vi "Bi-mode_VI_modified.vi"() -> ()   [LabVIEW 2014]
doc: "This VI demonstrates the individual configuration of settings in I/W, W/I, and continuous operation modes.\n\nThis VI is not meant to be used with infusion-only models. \n\nNotes:\n(1) If continuous mode is selected, infuse volumes/rates will be used."
uses:
  <instrlib>/KD Scientific 2XX Series/KD Scientific 2XX Series.lvlib
panel:
  out "Units":string
  out "Delivered Volume":dbl
  in  "stop":bool
  out "Status":T1
  in  "Baud Rate (9600)":u32(ring)=9600 items=["300"=300, "1200"=1200, "2400"=2400, "4800"=4800, "9600"=9600]
  in  "Withdrawal Settings":T2={"Flow Rate (5)"=5.0, "Volume (10)"=10.0, "Volume Units (ml)"=enum."milliliters (ml)", "Rate Units (ml/min.)"=enum."milliliters per minute (ml/min.)"} {"Volume (10)" format="%#.3g"}
  in  "Diameter (8.75 mm)":dbl=8.75
  in  "Infusion Settings":T2={"Flow Rate (5)"=5.0, "Volume (10)"=10.0, "Volume Units (ml)"=enum."milliliters (ml)", "Rate Units (ml/min.)"=enum."milliliters per minute (ml/min.)"}
  in  "Operation Mode (Infuse)":u16(ring) items=["Infuse", "Withdraw", "Infuse-Withdraw", "Withdraw-Infuse", "Continuous"]
  in  "Address (0)":i32 format="%0.0f"
  in  "error in (no error)":errorcluster
  in  "VISA resource name":refnum<visa-resource-name>="COM1"
  # "© 2005 National Instruments Corporation.  ALL RIGHTS RESERVED."
  # "RS-232 Settings"
  # "General Settings"
  # "Pump Status"
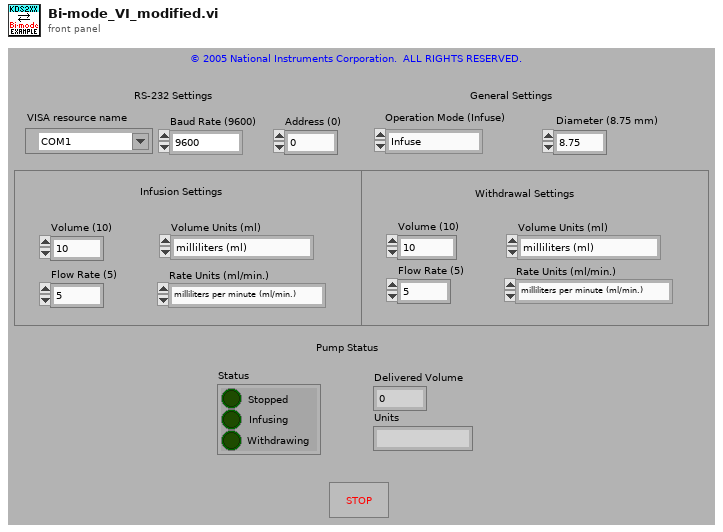
[diagram p1: front panel]
types:
  T1 = cluster{"Stopped":bool, "Infusing":bool, "Withdrawing":bool}
  T2 = cluster{"Flow Rate (5)":dbl, "Volume (10)":dbl, "Volume Units (ml)":enum16{"milliliters (ml)", "microliters (ul)"}, "Rate Units (ml/min.)":enum16{"milliliters per minute (ml/min.)", "milliliters per hour (ml/hr.)", "microliters per minute (ul/min.)", "microliters per hour (ul/hr.)"}}
  T3 = enum16{"milliliters per minute (ml/min.)", "milliliters per hour (ml/hr.)", "microliters per minute (ul/min.)", "microliters per hour (ul/hr.)"}
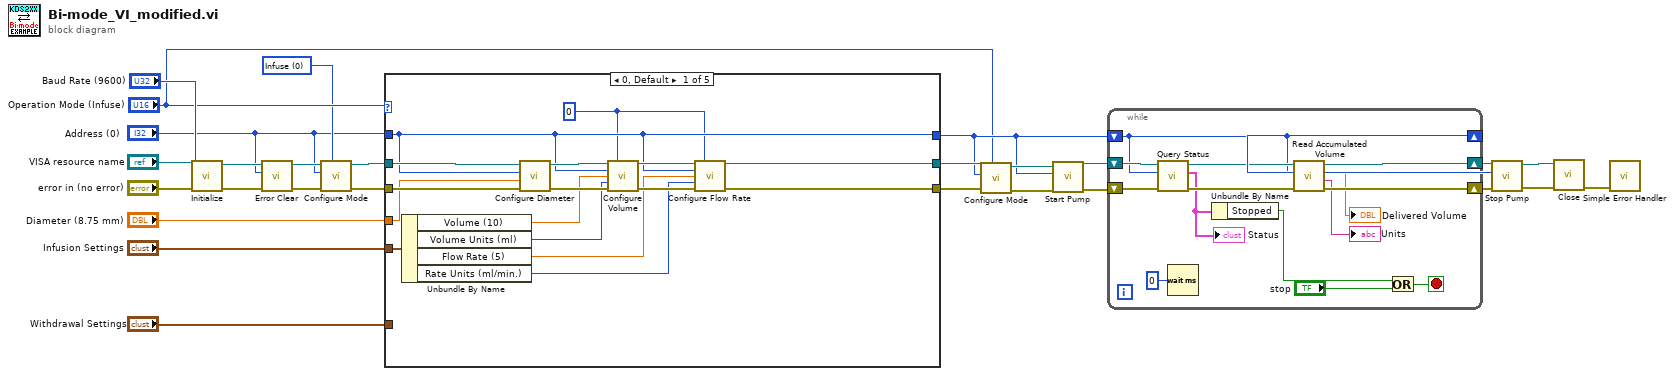
[diagram p0: block diagram]
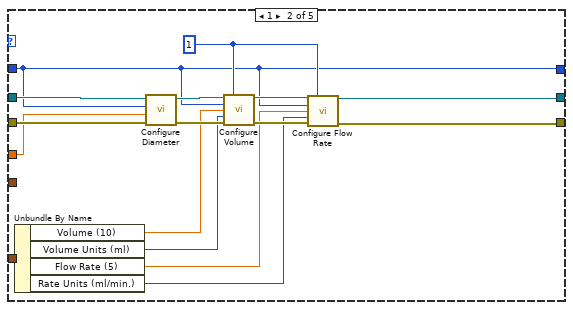
[diagram p2: hidden frame]
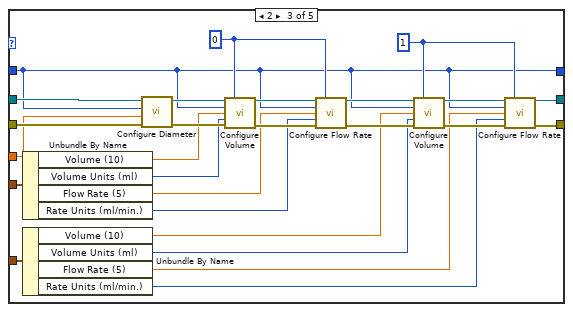
[diagram p3: hidden frame]
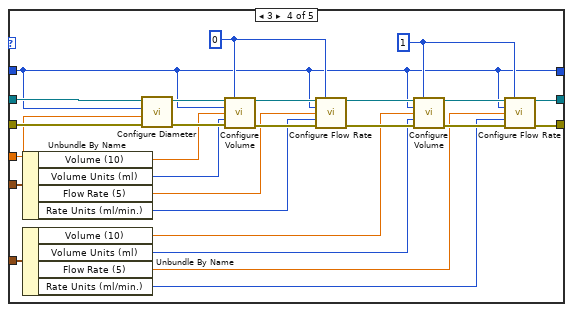
[diagram p4: hidden frame]
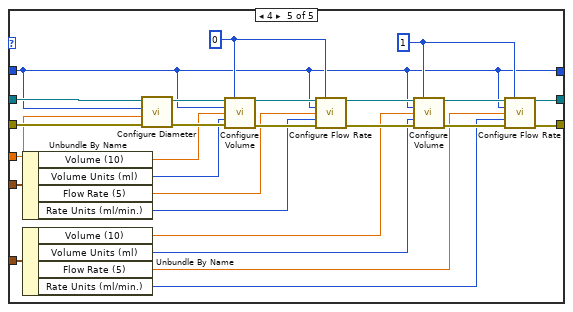
[diagram p5: hidden frame]
diagram:
  w6 = u16 0 items=["Infuse", "Withdraw", "Infuse-Withdraw", "Withdraw-Infuse", "Continuous"] ("Mode (infuse)")
  n1 = call <instrlib>:"Initialize.vi"("error in (no error)"="error in (no error)", "Baud Rate (9600)"="Baud Rate (9600)", "VISA resource name"="VISA resource name") -> ("error out"=w3:errorcluster, "VISA resource name out"=w2:refnum<visa-resource-name>)  [unwired: 7 in]
  n2 = call <instrlib>:"Error Clear.vi"("error in (no error)"=w3, "Address (0)"="Address (0)", "VISA resource name"=w2) -> ("error out"=w4:errorcluster, "VISA resource name out"=w5:refnum<visa-resource-name>)  [unwired: 6 in, 1 out]
  n3 = call <instrlib>:"Configure Mode.vi"("Mode (infuse)"=w6, "error in (no error)"=w4, "Address (0)"="Address (0)", "VISA resource name"=w5) -> ("error out"=w8:errorcluster, "VISA resource name out"=w7:refnum<visa-resource-name>)  [unwired: 6 in]
  n4 = case shown="0, Default" "Operation Mode (Infuse)" {
    tunnel: "Infusion Settings" -> [w38 _ w86 w112 w138]
    tunnel: "Withdrawal Settings" -> [_ w60 w85 w111 w137]
    tunnel: w7 -> [w44 w59 w84 w110 w136]
    tunnel: w8 -> [w43 w55 w83 w109 w135]
    tunnel: "Diameter (8.75 mm)" -> [w37 w51 w66 w92 w118]
    tunnel: [w36 w45 w61 w87 w113] -> w10
    tunnel: "Address (0)" -> [w36 w45 w61 w87 w113]
    tunnel: [w31 w56 w63 w89 w115] -> w14
    tunnel: [w30 w52 w62 w88 w114] -> w13
    frame 0, Default {
      w29 = 0
      n5 = Unbundle By Name(w38) -> ("Volume (10)"=w35:dbl, "Volume Units (ml)"=w34:enum16{"milliliters (ml)", "microliters (ul)"}, "Flow Rate (5)"=w33:dbl, "Rate Units (ml/min.)"=w32:T3)
      n6 = call <instrlib>:"Configure Diameter.vi"("error in (no error)"=w43, "Diameter (8.75 mm)"=w37, "Address (0)"=w36, "VISA resource name"=w44) -> ("error out"=w41:errorcluster, "VISA resource name out"=w42:refnum<visa-resource-name>)  [unwired: 6 in]
      n7 = call <instrlib>:"Configure Volume.vi"("VISA resource name"=w42, "Mode (infuse)"=w29, "Address (0)"=w36, "Volume (100)"=w35, "Units (0: milliliters)"=w34, "error in (no error)"=w41) -> ("VISA resource name out"=w40:refnum<visa-resource-name>, "error out"=w39:errorcluster)  [unwired: 8 in]
      n8 = call <instrlib>:"Configure Flow Rate.vi"("VISA resource name"=w40, "Mode (infuse)"=w29, "Address (0)"=w36, "Flow Rate (5)"=w33, "Units (0: milliliters per minute)"=w32, "error in (no error)"=w39) -> ("VISA resource name out"=w31:refnum<visa-resource-name>, "error out"=w30:errorcluster)  [unwired: 8 in]
    }
    frame 1 {
      w46 = 1
      n9 = Unbundle By Name(w60) -> ("Volume (10)"=w50:dbl, "Volume Units (ml)"=w49:enum16{"milliliters (ml)", "microliters (ul)"}, "Flow Rate (5)"=w48:dbl, "Rate Units (ml/min.)"=w47:T3)
      n10 = call <instrlib>:"Configure Diameter.vi"("error in (no error)"=w55, "Diameter (8.75 mm)"=w51, "Address (0)"=w45, "VISA resource name"=w59) -> ("error out"=w54:errorcluster, "VISA resource name out"=w58:refnum<visa-resource-name>)  [unwired: 6 in]
      n11 = call <instrlib>:"Configure Volume.vi"("VISA resource name"=w58, "Mode (infuse)"=w46, "Address (0)"=w45, "Volume (100)"=w50, "Units (0: milliliters)"=w49, "error in (no error)"=w54) -> ("VISA resource name out"=w57:refnum<visa-resource-name>, "error out"=w53:errorcluster)  [unwired: 8 in]
      n12 = call <instrlib>:"Configure Flow Rate.vi"("VISA resource name"=w57, "Mode (infuse)"=w46, "Address (0)"=w45, "Flow Rate (5)"=w48, "Units (0: milliliters per minute)"=w47, "error in (no error)"=w53) -> ("VISA resource name out"=w56:refnum<visa-resource-name>, "error out"=w52:errorcluster)  [unwired: 8 in]
    }
    frame 2 {
      w64 = 1
      w65 = 0
      n13 = Unbundle By Name(w86) -> ("Volume (10)"=w74:dbl, "Volume Units (ml)"=w73:enum16{"milliliters (ml)", "microliters (ul)"}, "Flow Rate (5)"=w72:dbl, "Rate Units (ml/min.)"=w71:T3)
      n14 = Unbundle By Name(w85) -> ("Volume (10)"=w70:dbl, "Volume Units (ml)"=w69:enum16{"milliliters (ml)", "microliters (ul)"}, "Flow Rate (5)"=w68:dbl, "Rate Units (ml/min.)"=w67:T3)
      n15 = call <instrlib>:"Configure Diameter.vi"("error in (no error)"=w83, "Diameter (8.75 mm)"=w66, "Address (0)"=w61, "VISA resource name"=w84) -> ("error out"=w78:errorcluster, "VISA resource name out"=w82:refnum<visa-resource-name>)  [unwired: 6 in]
      n16 = call <instrlib>:"Configure Volume.vi"("VISA resource name"=w82, "Mode (infuse)"=w65, "Address (0)"=w61, "Volume (100)"=w74, "Units (0: milliliters)"=w73, "error in (no error)"=w78) -> ("VISA resource name out"=w81:refnum<visa-resource-name>, "error out"=w77:errorcluster)  [unwired: 8 in]
      n17 = call <instrlib>:"Configure Flow Rate.vi"("VISA resource name"=w81, "Mode (infuse)"=w65, "Address (0)"=w61, "Flow Rate (5)"=w72, "Units (0: milliliters per minute)"=w71, "error in (no error)"=w77) -> ("VISA resource name out"=w80:refnum<visa-resource-name>, "error out"=w76:errorcluster)  [unwired: 8 in]
      n18 = call <instrlib>:"Configure Volume.vi"("VISA resource name"=w80, "Mode (infuse)"=w64, "Address (0)"=w61, "Volume (100)"=w70, "Units (0: milliliters)"=w69, "error in (no error)"=w76) -> ("VISA resource name out"=w79:refnum<visa-resource-name>, "error out"=w75:errorcluster)  [unwired: 8 in]
      n19 = call <instrlib>:"Configure Flow Rate.vi"("VISA resource name"=w79, "Mode (infuse)"=w64, "Address (0)"=w61, "Flow Rate (5)"=w68, "Units (0: milliliters per minute)"=w67, "error in (no error)"=w75) -> ("VISA resource name out"=w63:refnum<visa-resource-name>, "error out"=w62:errorcluster)  [unwired: 8 in]
    }
    frame 3 {
      w90 = 1
      w91 = 0
      n20 = Unbundle By Name(w112) -> ("Volume (10)"=w100:dbl, "Volume Units (ml)"=w99:enum16{"milliliters (ml)", "microliters (ul)"}, "Flow Rate (5)"=w98:dbl, "Rate Units (ml/min.)"=w97:T3)
      n21 = Unbundle By Name(w111) -> ("Volume (10)"=w96:dbl, "Volume Units (ml)"=w95:enum16{"milliliters (ml)", "microliters (ul)"}, "Flow Rate (5)"=w94:dbl, "Rate Units (ml/min.)"=w93:T3)
      n22 = call <instrlib>:"Configure Diameter.vi"("error in (no error)"=w109, "Diameter (8.75 mm)"=w92, "Address (0)"=w87, "VISA resource name"=w110) -> ("error out"=w104:errorcluster, "VISA resource name out"=w108:refnum<visa-resource-name>)  [unwired: 6 in]
      n23 = call <instrlib>:"Configure Volume.vi"("VISA resource name"=w108, "Mode (infuse)"=w91, "Address (0)"=w87, "Volume (100)"=w100, "Units (0: milliliters)"=w99, "error in (no error)"=w104) -> ("VISA resource name out"=w107:refnum<visa-resource-name>, "error out"=w103:errorcluster)  [unwired: 8 in]
      n24 = call <instrlib>:"Configure Flow Rate.vi"("VISA resource name"=w107, "Mode (infuse)"=w91, "Address (0)"=w87, "Flow Rate (5)"=w98, "Units (0: milliliters per minute)"=w97, "error in (no error)"=w103) -> ("VISA resource name out"=w106:refnum<visa-resource-name>, "error out"=w102:errorcluster)  [unwired: 8 in]
      n25 = call <instrlib>:"Configure Volume.vi"("VISA resource name"=w106, "Mode (infuse)"=w90, "Address (0)"=w87, "Volume (100)"=w96, "Units (0: milliliters)"=w95, "error in (no error)"=w102) -> ("VISA resource name out"=w105:refnum<visa-resource-name>, "error out"=w101:errorcluster)  [unwired: 8 in]
      n26 = call <instrlib>:"Configure Flow Rate.vi"("VISA resource name"=w105, "Mode (infuse)"=w90, "Address (0)"=w87, "Flow Rate (5)"=w94, "Units (0: milliliters per minute)"=w93, "error in (no error)"=w101) -> ("VISA resource name out"=w89:refnum<visa-resource-name>, "error out"=w88:errorcluster)  [unwired: 8 in]
    }
    frame 4 {
      w116 = 1
      w117 = 0
      n27 = Unbundle By Name(w138) -> ("Volume (10)"=w126:dbl, "Volume Units (ml)"=w125:enum16{"milliliters (ml)", "microliters (ul)"}, "Flow Rate (5)"=w124:dbl, "Rate Units (ml/min.)"=w123:T3)
      n28 = Unbundle By Name(w137) -> ("Volume (10)"=w122:dbl, "Volume Units (ml)"=w121:enum16{"milliliters (ml)", "microliters (ul)"}, "Flow Rate (5)"=w120:dbl, "Rate Units (ml/min.)"=w119:T3)
      n29 = call <instrlib>:"Configure Diameter.vi"("error in (no error)"=w135, "Diameter (8.75 mm)"=w118, "Address (0)"=w113, "VISA resource name"=w136) -> ("error out"=w130:errorcluster, "VISA resource name out"=w134:refnum<visa-resource-name>)  [unwired: 6 in]
      n30 = call <instrlib>:"Configure Volume.vi"("VISA resource name"=w134, "Mode (infuse)"=w117, "Address (0)"=w113, "Volume (100)"=w126, "Units (0: milliliters)"=w125, "error in (no error)"=w130) -> ("VISA resource name out"=w133:refnum<visa-resource-name>, "error out"=w129:errorcluster)  [unwired: 8 in]
      n31 = call <instrlib>:"Configure Flow Rate.vi"("VISA resource name"=w133, "Mode (infuse)"=w117, "Address (0)"=w113, "Flow Rate (5)"=w124, "Units (0: milliliters per minute)"=w123, "error in (no error)"=w129) -> ("VISA resource name out"=w132:refnum<visa-resource-name>, "error out"=w128:errorcluster)  [unwired: 8 in]
      n32 = call <instrlib>:"Configure Volume.vi"("VISA resource name"=w132, "Mode (infuse)"=w116, "Address (0)"=w113, "Volume (100)"=w122, "Units (0: milliliters)"=w121, "error in (no error)"=w128) -> ("VISA resource name out"=w131:refnum<visa-resource-name>, "error out"=w127:errorcluster)  [unwired: 8 in]
      n33 = call <instrlib>:"Configure Flow Rate.vi"("VISA resource name"=w131, "Mode (infuse)"=w116, "Address (0)"=w113, "Flow Rate (5)"=w120, "Units (0: milliliters per minute)"=w119, "error in (no error)"=w127) -> ("VISA resource name out"=w115:refnum<visa-resource-name>, "error out"=w114:errorcluster)  [unwired: 8 in]
    }
  }
  n34 = call <instrlib>:"Configure Mode.vi"("Mode (infuse)"="Operation Mode (Infuse)", "error in (no error)"=w13, "Address (0)"=w10, "VISA resource name"=w14) -> ("error out"=w11:errorcluster, "VISA resource name out"=w12:refnum<visa-resource-name>)  [unwired: 6 in]
  n35 = call <instrlib>:"Start Pump.vi"("error in (no error)"=w11, "Address (0)"=w10, "VISA resource name"=w12) -> ("error out"=w25:errorcluster, "VISA resource name out"=w26:refnum<visa-resource-name>)  [unwired: 7 in]
  n36 = while {
    shift-right: [w141] -> w19
    shift-left: w10 -> [w141]
    shift-right: [w143] -> w24
    shift-left: w26 -> [w149]
    shift-right: [w142] -> w23
    shift-left: w25 -> [w150]
    stop <- w147 stop-if-true
    n37 = call <instrlib>:"Query Status.vi"("error in (no error)"=w150, "Address (0)"=w141, "VISA resource name"=w149) -> ("error out"=w152:errorcluster, "Status"=w148:T1, "VISA resource name out"=w144:refnum<visa-resource-name>)  [unwired: 6 in]
    "Status" <- w148
    n38 = Wait (ms)(milliseconds to wait=u32 0) -> ()  [unwired: 1 out]
    n39 = Unbundle By Name(w148) -> ("Stopped"=w146:bool)
    n40 = call <instrlib>:"Read Accumulated Volume.vi"("error in (no error)"=w152, "Address (0)"=w141, "VISA resource name"=w144) -> ("error out"=w142:errorcluster, "Units"=→"Units":string, "Delivered Volume"=→"Delivered Volume":dbl, "VISA resource name out"=w143:refnum<visa-resource-name>)  [unwired: 5 in]
    n41 = Or(x=w146, y="stop") -> (x .or. y?=w147:bool)
  }
  n42 = call <instrlib>:"Stop Pump.vi"("error in (no error)"=w23, "Address (0)"=w19, "VISA resource name"=w24) -> ("error out"=w17:errorcluster, "VISA resource name out"=w16:refnum<visa-resource-name>)  [unwired: 7 in]
  n43 = call <instrlib>:"Close.vi"("error in (no error)"=w17, "VISA resource name"=w16) -> ("error out"=w18:errorcluster)  [unwired: 9 in]
  n44 = call <vilib>:"Simple Error Handler.vi"("error in (no error)"=w18) -> ()  [unwired: 4 in, 5 out]
